vi "Position Restrictions.vi"(4 "Pole Height\nfrom ground":dbl, 6 "Robot Height":dbl, 7 "Robot Width":dbl, 8 "Forearm Length":dbl, 9 "Backarm Length":dbl, 10 "newY":dbl, 11 "newX":dbl) -> (2 "modified Y":dbl, 3 "modified X":dbl)   [LabVIEW 2017]
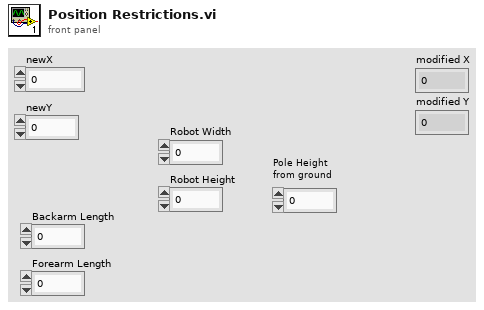
[diagram p1: front panel]
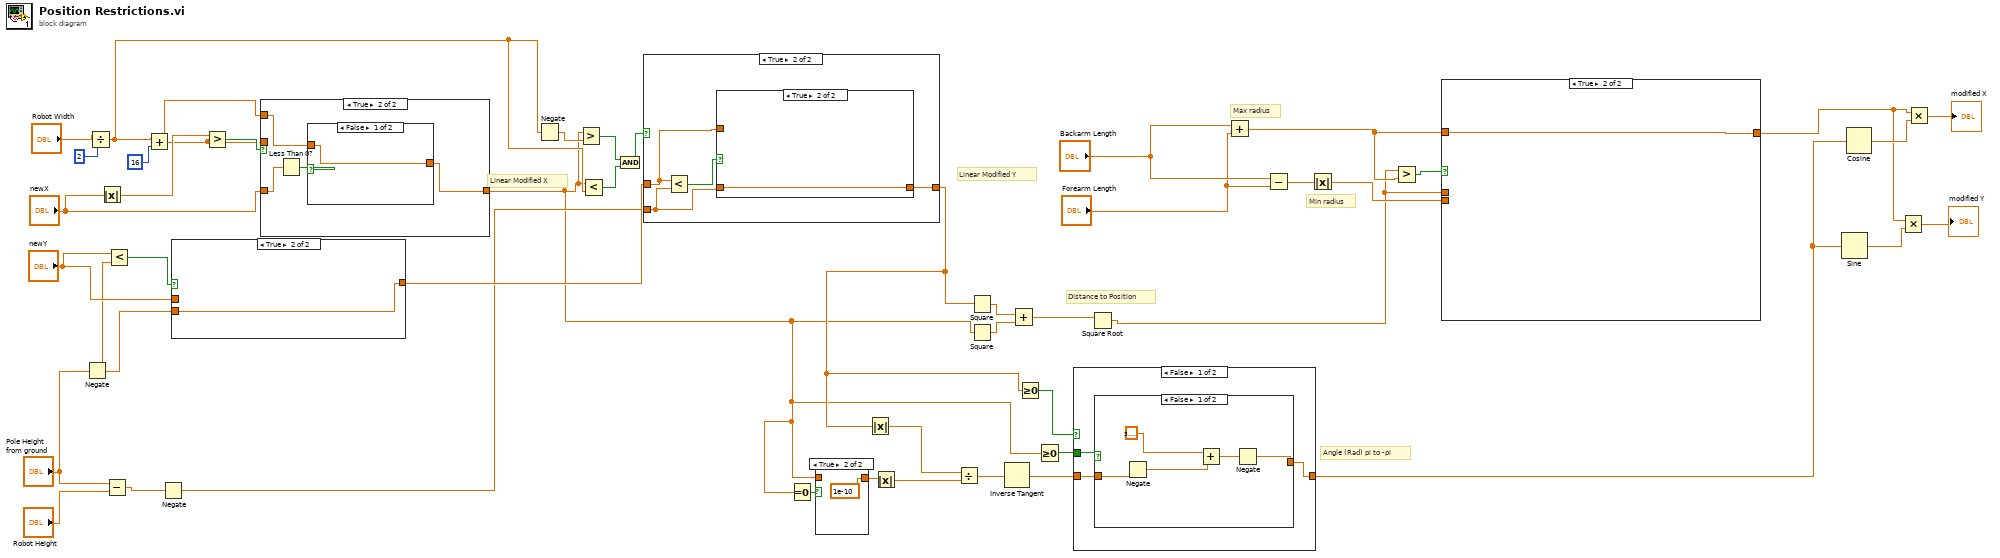
[diagram p0: block diagram]
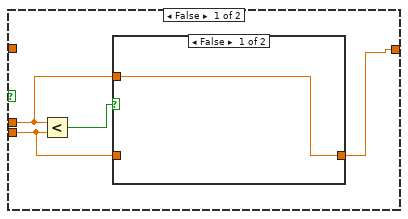
[diagram p3: hidden frame]
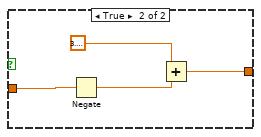
[diagram p5: hidden frame]
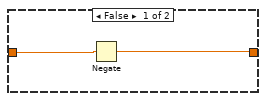
[diagram p7: hidden frame]
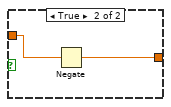
[diagram p12: hidden frame]
diagram:
  # "Min radius"
  # "Max radius"
  # "Angle (Rad) pi to -pi"
  # "Distance to Position"
  # "Linear Modified Y"
  # "Linear Modified X"
  n1 = Negate(x="Pole Height\nfrom ground") -> (-x=w1:dbl)
  n2 = Divide(x="Robot Width", y=2) -> (x/y=w38:dbl)
  n3 = Absolute Value(x="newX") -> (abs(x)=w42:dbl)
  n4 = Subtract(x="Pole Height\nfrom ground", y="Robot Height") -> (x-y=w32:dbl)
  n5 = Less?(x="newY", y=w1) -> (x < y?=w2:bool)
  n6 = Add(x=w38, y=16) -> (x+y=w40:dbl)
  n7 = Negate(x=w32) -> (-x=w31:dbl)
  n8 = case shown="True" w2 {
    tunnel: [w47 w48] -> w34
    tunnel: "newY" -> [w47 _]
    tunnel: w1 -> [_ w48]
    frame False {
    }
    frame True {
    }
  }
  n9 = Greater?(x=w42, y=w40) -> (0:w43:bool)
  n10 = case shown="True" w43 {
    tunnel: w40 -> [_ _]
    tunnel: "newX" -> [w49 w53]
    tunnel: [w49 w50] -> w5
    tunnel: w40 -> [_ w51]
    frame False {
    }
    frame True {
      n11 = Less Than 0?(x=w53) -> (x < 0?=w52:bool)
      n12 = case shown="False" w52 {
        tunnel: w51 -> [w54 w56]
        tunnel: [w54 w55] -> w50
        frame False {
        }
        frame True {
          n13 = Negate(x=w56) -> (-x=w55:dbl)
        }
      }
    }
  }
  n14 = Negate(x=w38) -> (-x=w39:dbl)
  n15 = Greater?(x=w5, y=w39) -> (0:w37:bool)
  n16 = Less?(x=w5, y=w38) -> (x < y?=w36:bool)
  n17 = And(x=w37, y=w36) -> (x .and. y?=w35:bool)
  n18 = case shown="True" w35 {
    tunnel: w34 -> [w57 w59]
    tunnel: w31 -> [_ w60]
    tunnel: [w57 w58] -> w21
    frame False {
    }
    frame True {
      n19 = Less?(x=w59, y=w60) -> (x < y?=w61:bool)
      n20 = case shown="True" w61 {
        tunnel: w60 -> [_ w63]
        tunnel: [w62 w63] -> w58
        tunnel: w59 -> [w62 _]
        frame False {
        }
        frame True {
        }
      }
    }
  }
  n21 = Equal To 0?(x=w5) -> (x = 0?=w7:bool)
  n22 = case shown="True" w7 {
    tunnel: [w64 1e-10] -> w6
    tunnel: w5 -> [w64 _]
    frame False {
    }
    frame True {
    }
  }
  n23 = Absolute Value(x=w21) -> (abs(x)=w27:dbl)
  n24 = Absolute Value(x=w6) -> (abs(x)=w26:dbl)
  n25 = Divide(x=w27, y=w26) -> (x/y=w25:dbl)
  n26 = Square(x=w21) -> (x^2=w30:dbl)
  n27 = Square(x=w5) -> (x^2=w29:dbl)
  n28 = Inverse Tangent(1:w25) -> (0:w22:dbl)
  n29 = Add(x=w30, y=w29) -> (x+y=w28:dbl)
  n30 = Greater Or Equal To 0?(x=w21) -> (x >= 0?=w24:bool)
  n31 = Greater Or Equal To 0?(x=w5) -> (x >= 0?=w23:bool)
  n32 = case shown="False" w24 {
    tunnel: w23 -> [w68 w80]
    tunnel: w22 -> [w67 w79]
    tunnel: [w66 w78] -> w13
    frame False {
      n33 = case shown="False" w68 {
        tunnel: w67 -> [w71 w77]
        tunnel: [w69 w74] -> w66
        frame False {
          n34 = Negate(x=w71) -> (-x=w73:dbl)
          n35 = Add(x=3.141592653589793, y=w73) -> (x+y=w70:dbl)
          n36 = Negate(x=w70) -> (-x=w69:dbl)
        }
        frame True {
          n37 = Negate(x=w77) -> (-x=w75:dbl)
          n38 = Add(x=3.141592653589793, y=w75) -> (x+y=w74:dbl)
        }
      }
    }
    frame True {
      n39 = case shown="True" w80 {
        tunnel: w79 -> [w82 w83]
        tunnel: [w81 w83] -> w78
        frame False {
          n40 = Negate(x=w82) -> (-x=w81:dbl)
        }
        frame True {
        }
      }
    }
  }
  n41 = Square Root(x=w28) -> (sqrt(x)=w14:dbl)
  n42 = Add(x="Backarm Length", y="Forearm Length") -> (x+y=w16:dbl)
  n43 = Subtract(x="Backarm Length", y="Forearm Length") -> (x-y=w18:dbl)
  n44 = Absolute Value(x=w18) -> (abs(x)=w15:dbl)
  n45 = Greater?(x=w14, y=w16) -> (0:w17:bool)
  n46 = case shown="True" w17 {
    tunnel: [w85 w90] -> w11
    tunnel: w16 -> [_ w90]
    tunnel: w15 -> [w86 _]
    tunnel: w14 -> [w84 _]
    frame False {
      n47 = Less?(x=w84, y=w86) -> (x < y?=w87:bool)
      n48 = case shown="False" w87 {
        tunnel: w86 -> [_ w89]
        tunnel: [w88 w89] -> w85
        tunnel: w84 -> [w88 _]
        frame False {
        }
        frame True {
        }
      }
    }
    frame True {
    }
  }
  n49 = Sine(x=w13) -> (sin(x)=w10:dbl)
  n50 = Cosine(x=w13) -> (cos(x)=w12:dbl)
  n51 = Multiply(x=w11, y=w10) -> (x*y=→"modified Y":dbl)
  n52 = Multiply(x=w11, y=w12) -> (x*y=→"modified X":dbl)
